vi "main.vi"() -> ()   [LabVIEW 2023]
uses:
  <vilib>/vision/Image Controls.llb/IMAQ Image.ctl
  <vilib>/vision/NI_Vision_Development_Module.lvlib
  <vilib>/vision/Pattern Matching.llb/IMAQ Match Range Setting.ctl
  <vilib>/vision/Shape Detection.llb/ShapeDetectionMatchOptions.ctl
  <vilib>/addons/database/NI_Database_API.lvlib
  <vilib>/addons/database/Command.llb/Cmd Set Parameter Value (C).vi
  <vilib>/addons/database/Command.llb/Cmd Delete.vi
  <vilib>/addons/database/Recordset.llb/Rec Destroy - Command.vi
  <vilib>/addons/database/Command.llb/Cmd Execute.vi
  <vilib>/addons/database/Connection.llb/DB Tools Open Connec (String).vi
  <vilib>/Utility/error.llb/DialogType.ctl
panel:
  in  "Python":bool
  out "Triangles":i32
  out "String":string
  out "Rectangles":i32
  out "Circles":i32
  out "Obraz":T1(plugin-control)
  in  "Output Path":path
  in  "Input Path":path=path "C:/Users/kacpe/Desktop/OSP/testp.png"
  in  "Refresh Button":bool
  in  "Process Stop Button":bool
  in  "Save As Button":bool
  in  "Labview":bool
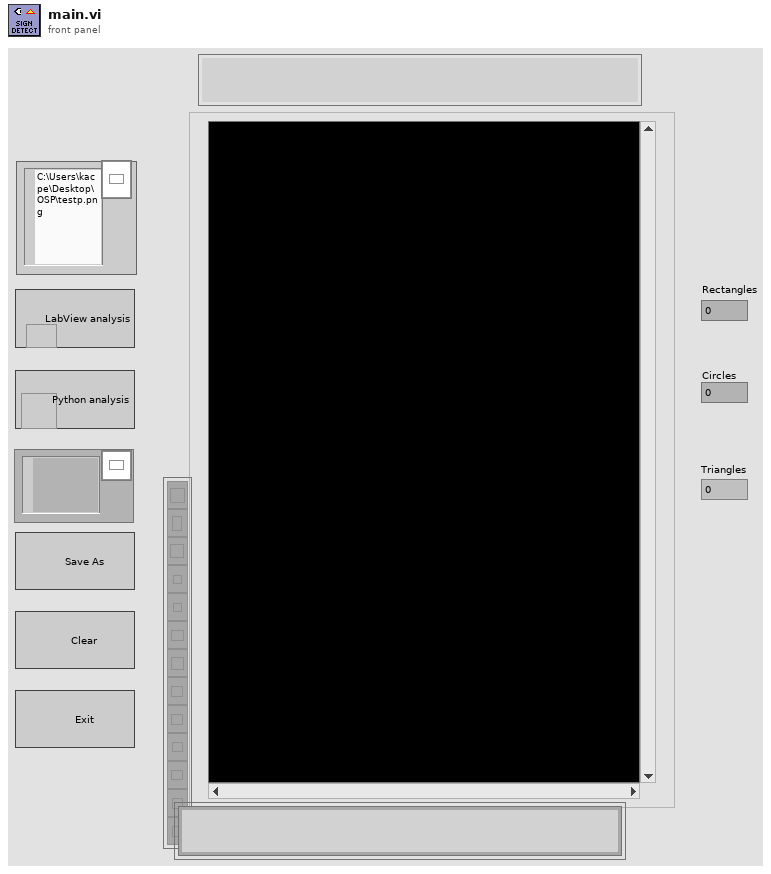
[diagram p1: front panel]
types:
  T1 = typedef "IMAQ Image.ctl" = refnum<image>
  T2 = enum32{"Invalid", "Standard", "Closed", "Hidden", "Minimized", "Maximized"}
  T3 = enum32{"invalid app kind", "Development System", "Run Time System", "Student Edition", "Embedded LabVIEW", "Evaluation", "Custom"}
  T4 = cluster{"Position":cluster{"x":sgl, "y":sgl}, "Angle":sgl, "Scale":sgl, "Score":sgl, "Bounding Box":cluster{"x":sgl, "y":sgl}[]}[]
  T5 = cluster{"Left":i32, "Top":i32, "Right":i32, "Bottom":i32}
  T6 = cluster{"Corners":cluster{"X":sgl, "Y":sgl}[], "Angle":dbl, "Width":dbl, "Height":dbl, "Score":dbl}[]
  T7 = cluster{"Position":cluster{"X":sgl, "Y":sgl}, "Radius":dbl, "Score":dbl}[]
  T8 = cluster{"Min Width":dbl, "Max Width":dbl, "Min Height":dbl, "Max Height":dbl}
  T9 = cluster{"Core":cluster{"Current VI Reference":refnum<vi>, "Close Panel on Exit?":bool}, "Obraz":T1, enum16{"null", "kwadrat", "kolo", "trojkat"}, "Rectangles":cluster{"Corners":cluster{"X":sgl, "Y":sgl}[], "Angle":dbl, "Width":dbl, "Height":dbl, "Score":dbl}[], "Circles":cluster{"Position":cluster{"X":sgl, "Y":sgl}, "Radius":dbl, "Score":dbl}[], "Triangle":cluster{"Position":cluster{"x":sgl, "y":sgl}, "Angle":sgl, "Scale":sgl, "Score":sgl, "Bounding Box":cluster{"x":sgl, "y":sgl}[]}[], "Znak":string, "Input Path":path, "Python cords":cluster{"Left":i32, "Top":i32, "Right":i32, "Bottom":i32}, "L/p":string}
  T10 = typedef "DialogType.ctl" = u16
  T11 = cluster{"Current VI Reference":refnum<vi>, "Close Panel on Exit?":bool}
  T12 = typedef "ShapeDetectionMatchOptions.ctl" = cluster{"Rotation":bool, "Scale":bool, "Occlusion":bool, "Range Settings":T13[]}
  T13 = typedef "IMAQ Match Range Setting.ctl" = cluster{"Match Constraints":u32, "Min":dbl, "Max":dbl}
  T14 = typedef "Image Type" = u32
  T15 = typedef "NI_Database_API.lvlib/Conn ObjectReference.ctl" = refnum<k1>
  T16 = typedef "NI_Database_API.lvlib/Cmd ObjectReference.ctl" = refnum<k1>
  T17 = typedef "NI_Database_API.lvlib/Cmd-Rec Object Reference.ctl" = refnum<k1>
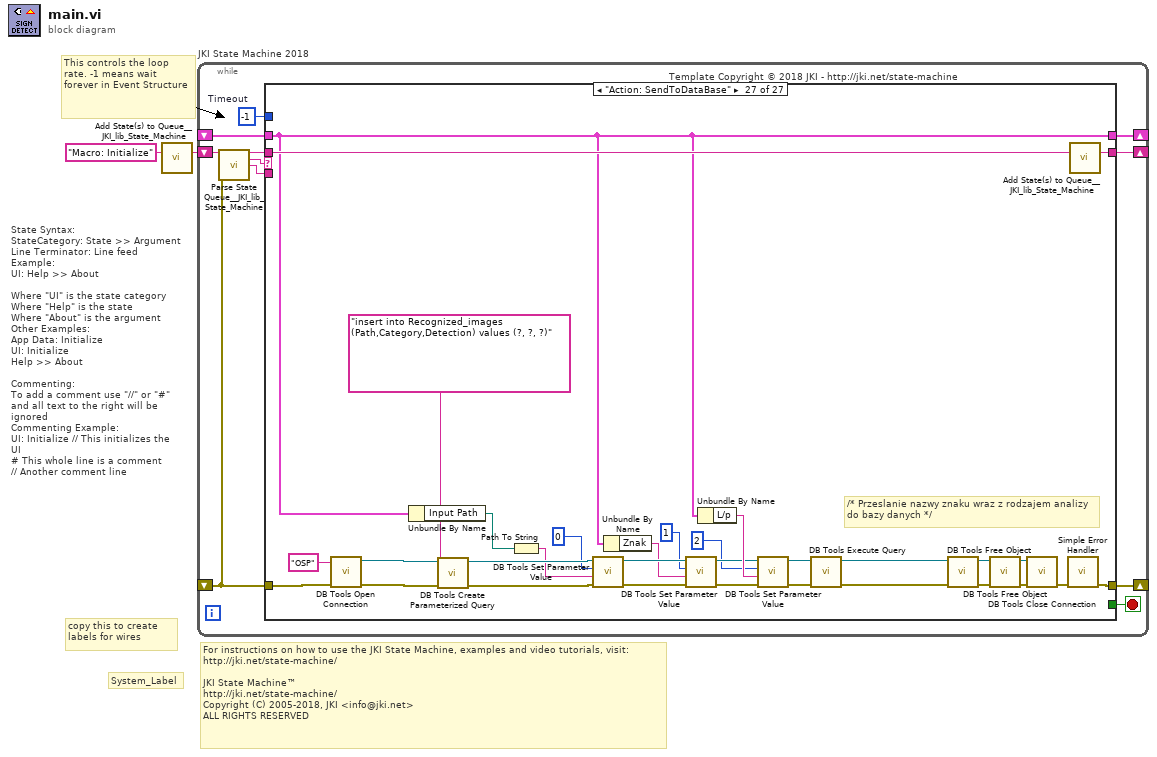
[diagram p0: block diagram]
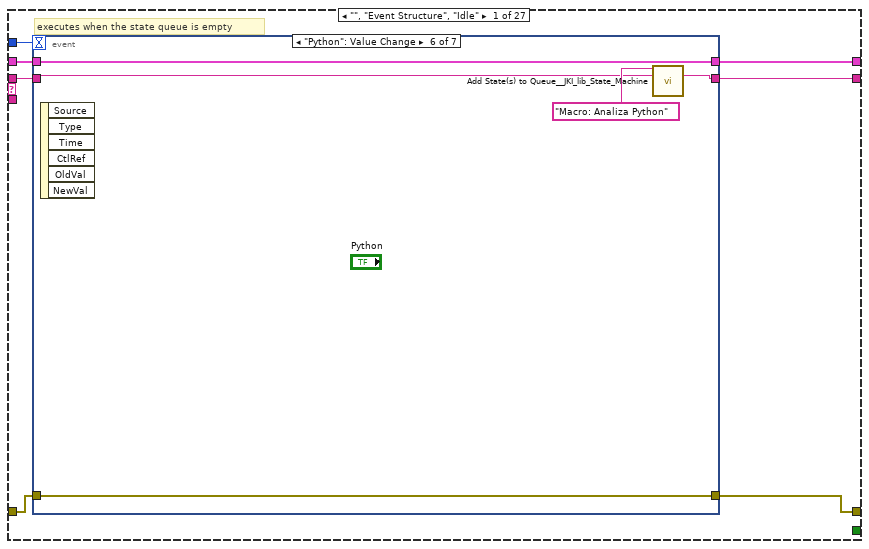
[diagram p2: hidden frame]
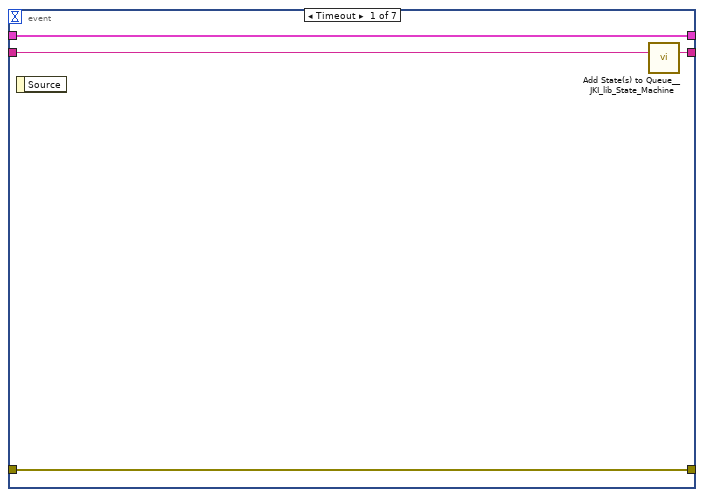
[diagram p3: hidden frame]
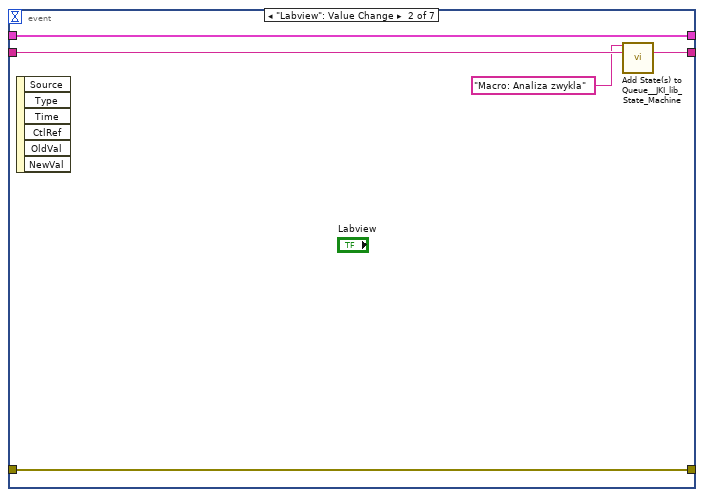
[diagram p4: hidden frame]
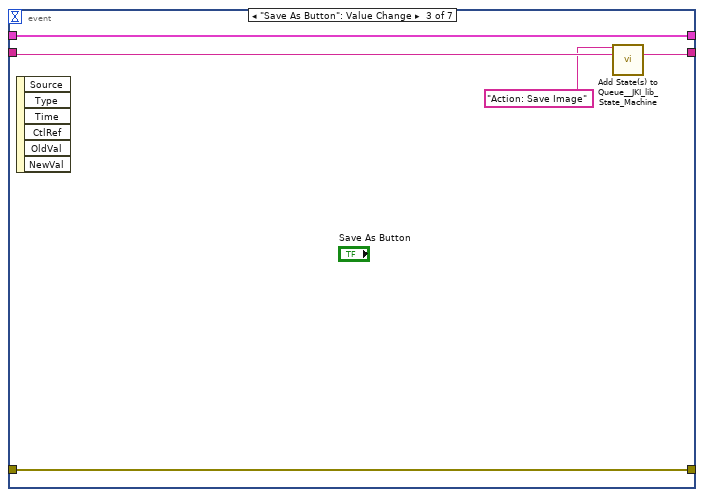
[diagram p5: hidden frame]
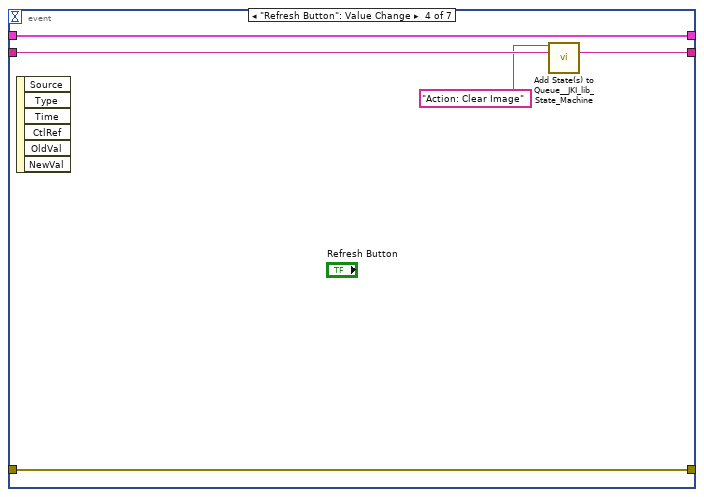
[diagram p6: hidden frame]
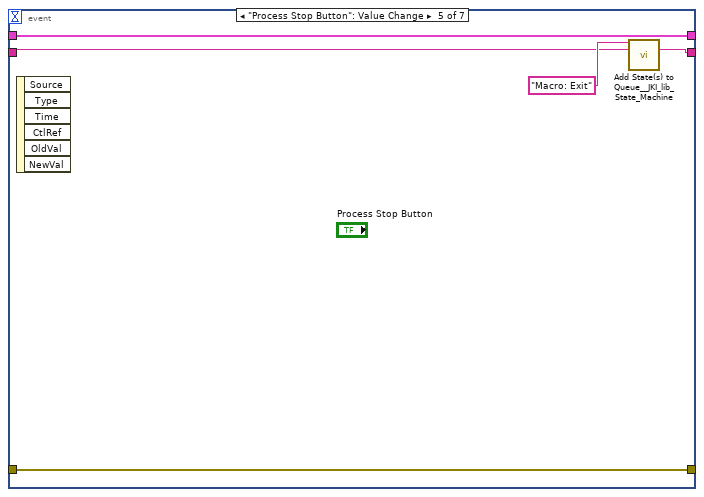
[diagram p7: hidden frame]
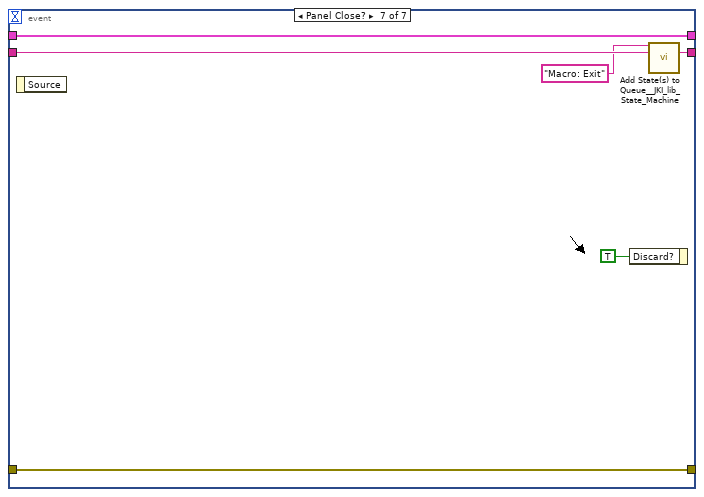
[diagram p8: hidden frame]
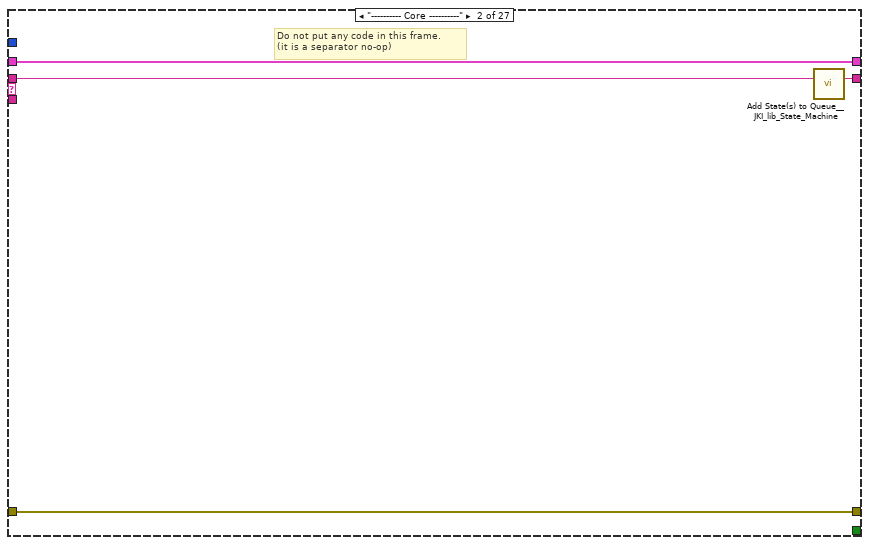
[diagram p9: hidden frame]
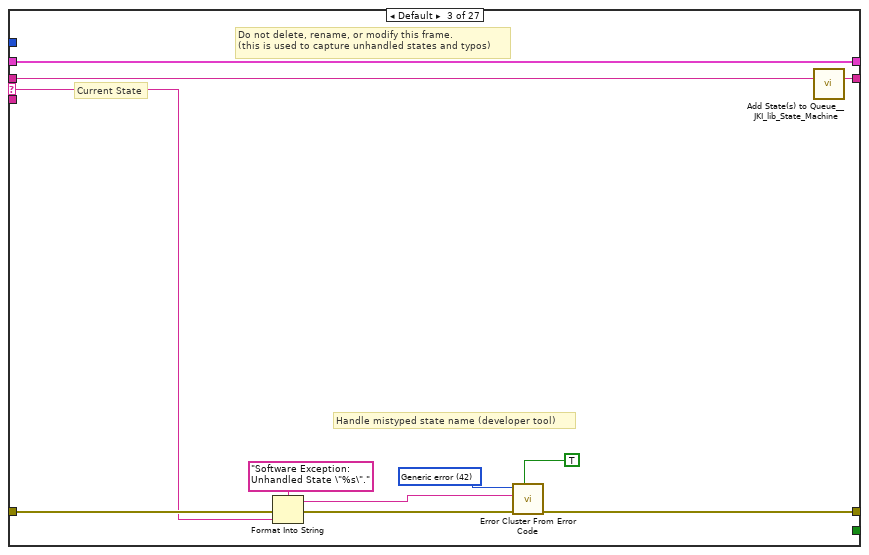
[diagram p10: hidden frame]
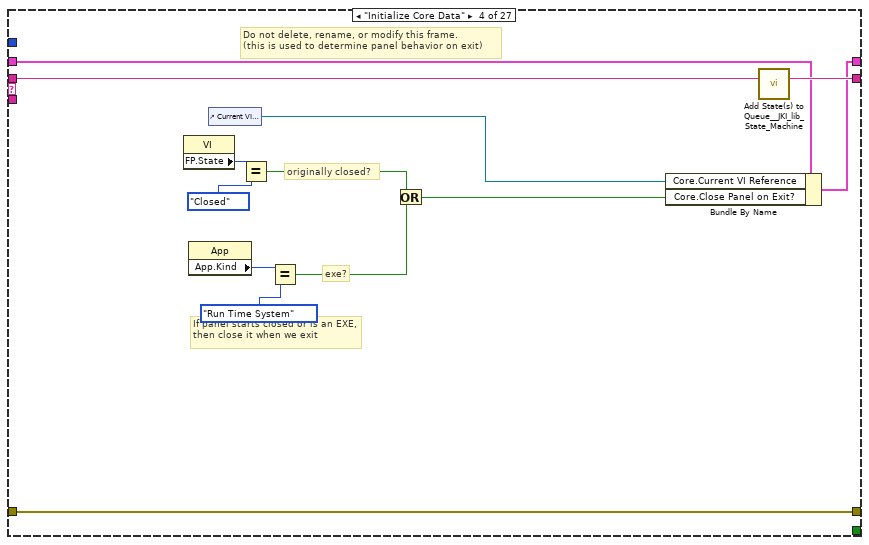
[diagram p11: hidden frame]
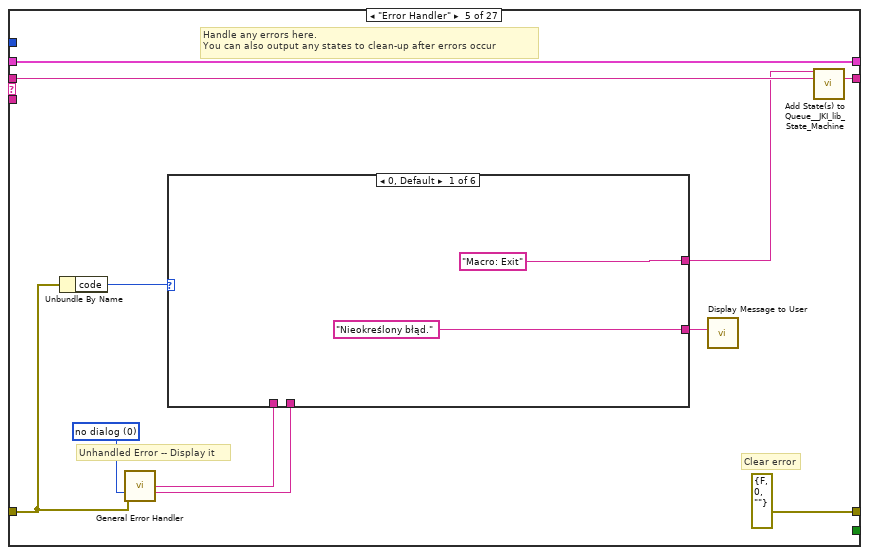
[diagram p12: hidden frame]
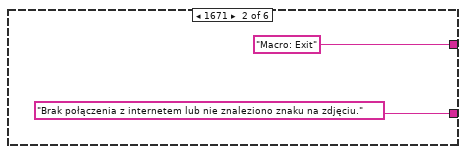
[diagram p13: hidden frame]
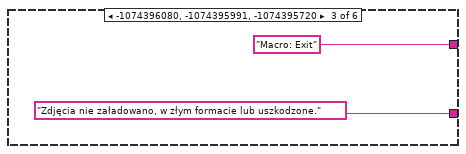
[diagram p14: hidden frame]
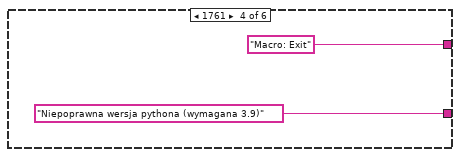
[diagram p15: hidden frame]
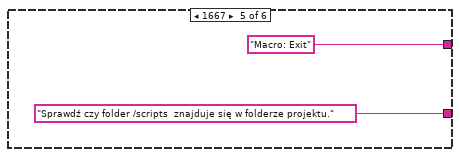
[diagram p16: hidden frame]
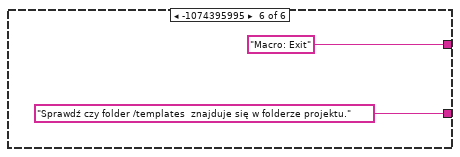
[diagram p17: hidden frame]
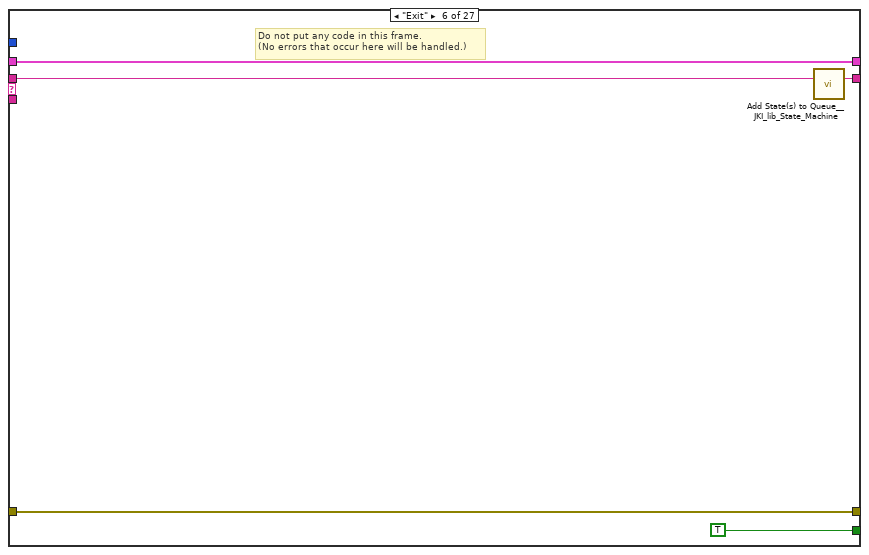
[diagram p18: hidden frame]
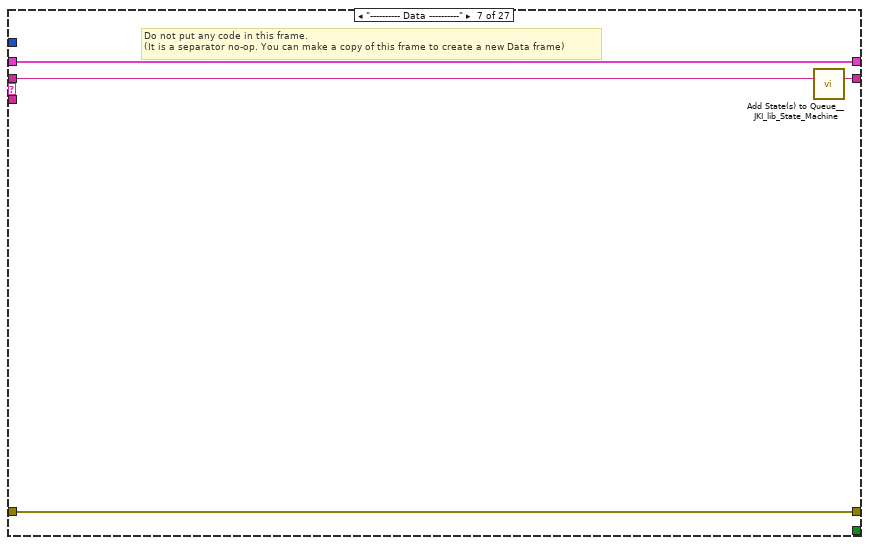
[diagram p19: hidden frame]
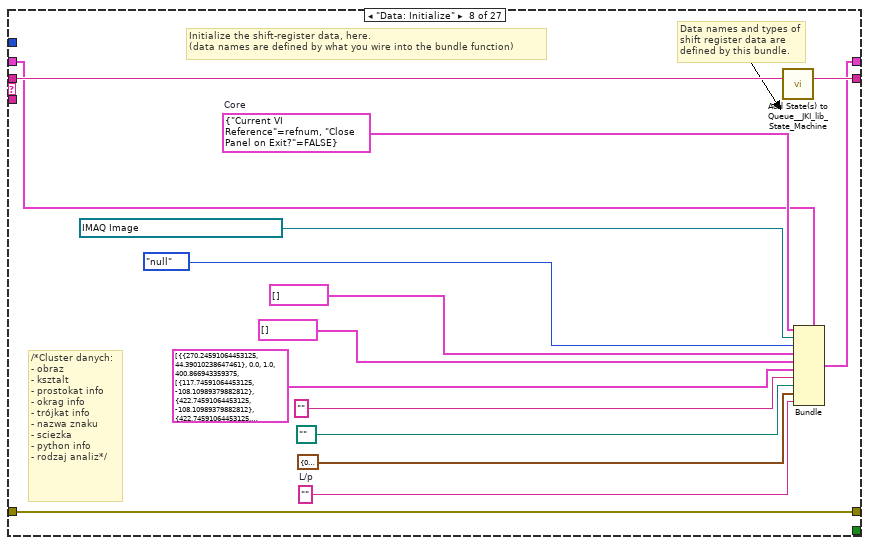
[diagram p20: hidden frame]
diagram:
  # "For instructions on how to use the JKI State Machine, examples and video tutorials, visit:\nhttp://jki.net/state-machine/\n\nJKI State Machine™\nhttp://jki.net/state-machine/\nCopyright (C) 2005-2018, JKI <info@jki.net>\nALL RIGHTS RESERVED"
  # "State Syntax:\nStateCategory: State >> Argument\nLine Terminator: Line feed\nExample:\nUI: Help >> About\n\nWhere \"UI\" is the state category\nWhere \"Help\" is the state\nWhere \"About\" is the argument\nOther Examples:\nApp Data: Initialize\nUI: Initialize\nHelp >> About\n\nCommenting:\nTo add a comment use \"//\" or \"#\" and all text to the right will be ignored\nCommenting Example:\nUI: Initialize // This initializes the UI\n# This whole line is a comment\n// Another comment line"
  # "copy this to create labels for wires"
  # "This controls the loop rate. -1 means wait forever in Event Structure"
  # "System_Label"
  n1 = call <vilib>:"Add State(s) to Queue__JKI_lib_State_Machine.vi"("State(s) in (\"\")"="Macro: Initialize") -> ("States Out"=w2:string)  [unwired: 14 in]
  n2 = while "JKI State Machine 2018" {
    shift-right: [w6] -> _
    shift-left: _ -> [w5]
    shift-right: [w9] -> _
    shift-left: _ -> [w3]
    shift-right: [w8] -> _
    shift-left: w2 -> [w10]
    stop <- w7 stop-if-true
    w4 = -1  # Timeout
    # "Template Copyright © 2018 JKI - http://jki.net/state-machine"
    n3 = call <vilib>:"Parse State Queue__JKI_lib_State_Machine.vi"("State Queue"=w10, "Error In (no error)"=w3) -> ("Remaining States"=w12:string, "Current State"=w13:string, "Arguments"=w11:string)  [unwired: 11 in]
    n4 = case shown="\"Action: SendToDataBase\"" w13 {
      selector: w13 -> [_ _ w60 _ _ _ _ _ _ _ _ _ _ _ _ _ _ _ _ _ _ _ _ _ _ _ _]
      tunnel: w12 -> [w20 w59 w64 w83 w94 w111 w115 w130 w136 w140 w144 w149 w155 w166 w230 w235 w240 w245 w255 w259 w298 w313 w344 w354 w361 w369 w400]
      tunnel: w11 -> [_ _ _ _ _ _ _ _ _ _ _ _ w150 w161 _ _ _ _ _ _ _ _ _ _ _ _ _]
      tunnel: w5 -> [w18 w56 w62 w72 w91 w109 w112 w119 w132 w137 w143 w147 w153 w160 w227 w232 w237 w242 w247 w256 w287 w307 w327 w346 w356 w364 w381]
      tunnel: [w17 w57 w66 w81 errorcluster {"status"=FALSE, "code"=0, "source"=""} ("error out") w108 w113 w128 w133 w138 w145 w146 w151 w163 w228 w233 w238 w243 w253 w257 w265 w311 w342 w349 w359 w367 w374] -> w9
      tunnel: w3 -> [w16 w57 w65 w81 w87 w108 w113 w128 w134 w138 w145 w146 w152 w164 w228 w233 w238 w243 w253 w257 w291 w310 w341 w349 w358 w367 w373]
      tunnel: [w19 w58 w63 w82 w93 w110 w114 w129 w135 w139 w144 w148 w154 w165 w229 w234 w239 w244 w254 w258 w298 w312 w343 w353 w360 w368 w399] -> w8
      tunnel: [_ _ _ _ _ TRUE _ _ _ _ _ _ _ _ _ _ _ _ _ _ _ _ _ _ _ _ _] -> w7
      tunnel: [w15 w56 w62 w71 w91 w109 w112 w118 w132 w137 w143 w147 w153 w160 w227 w232 w237 w242 w247 w256 w288 w308 w328 w347 w356 w365 w381] -> w6
      tunnel: w4 -> [w14 _ _ _ _ _ _ _ _ _ _ _ _ _ _ _ _ _ _ _ _ _ _ _ _ _ _]
      frame "", "Event Structure", "Idle" {
        # "executes when the state queue is empty"
        n5 = event shown="[5] \"Python\": Value Change" {
          selector: _ -> [_ _ _ _ _ _ _]
          dyn-events: _ -> [_ _ _ _ _ _ _]
          timeout: w14 -> [_ _ _ _ _ _ _]
          tunnel: w20 -> [w24 w27 w31 w36 w41 w46 w55]
          tunnel: [w23 w28 w32 w37 w43 w48 w54] -> w19
          tunnel: w18 -> [w21 w29 w34 w39 w44 w49 w52]
          tunnel: [w22 w25 w33 w38 w40 w45 w53] -> w17
          tunnel: w16 -> [w22 w25 w33 w38 w40 w45 w53]
          tunnel: [w21 w29 w34 w39 w44 w49 w52] -> w15
          event Timeout {
            n6 = event-data() -> ()  [unwired: 1 in, 1 out]
            n7 = call <vilib>:"Add State(s) to Queue__JKI_lib_State_Machine.vi"("State(s) in (\"\")"=w24) -> ("States Out"=w23:string)  [unwired: 14 in]
          }
          event "Labview": Value Change {
            n8 = event-data() -> ()  [unwired: 1 in, 6 out]
            n9 = call <vilib>:"Add State(s) to Queue__JKI_lib_State_Machine.vi"("State(s) in Front (\"\")"="Macro: Analiza zwykla" ("State(s) in Front (\"\")"), "State(s) in (\"\")"=w27) -> ("States Out"=w28:string)  [unwired: 13 in]
          }
          event "Save As Button": Value Change {
            n10 = event-data() -> ()  [unwired: 1 in, 6 out]
            n11 = call <vilib>:"Add State(s) to Queue__JKI_lib_State_Machine.vi"("State(s) in Front (\"\")"="Action: Save Image" ("State(s) in Front (\"\")"), "State(s) in (\"\")"=w31) -> ("States Out"=w32:string)  [unwired: 13 in]
          }
          event "Refresh Button": Value Change {
            n12 = event-data() -> ()  [unwired: 1 in, 6 out]
            n13 = call <vilib>:"Add State(s) to Queue__JKI_lib_State_Machine.vi"("State(s) in Front (\"\")"="Action: Clear Image" ("State(s) in Front (\"\")"), "State(s) in (\"\")"=w36) -> ("States Out"=w37:string)  [unwired: 13 in]
          }
          event "Process Stop Button": Value Change {
            n14 = event-data() -> ()  [unwired: 1 in, 6 out]
            n15 = call <vilib>:"Add State(s) to Queue__JKI_lib_State_Machine.vi"("State(s) in Front (\"\")"="Macro: Exit", "State(s) in (\"\")"=w41) -> ("States Out"=w43:string)  [unwired: 13 in]
          }
          event "Python": Value Change {
            n16 = event-data() -> ()  [unwired: 1 in, 6 out]
            n17 = call <vilib>:"Add State(s) to Queue__JKI_lib_State_Machine.vi"("State(s) in Front (\"\")"="Macro: Analiza Python", "State(s) in (\"\")"=w46) -> ("States Out"=w48:string)  [unwired: 13 in]
          }
          event Panel Close? {
            n18 = event-data() -> ()  [unwired: 1 in, 1 out]
            n19 = event-data ("Event Filter Node")("Discard?"=TRUE) -> ()  [unwired: 1 in, 1 out]
            n20 = call <vilib>:"Add State(s) to Queue__JKI_lib_State_Machine.vi"("State(s) in Front (\"\")"="Macro: Exit", "State(s) in (\"\")"=w55) -> ("States Out"=w54:string)  [unwired: 13 in]
          }
        }
      }
      frame "---------- Core ----------" {
        # "Do not put any code in this frame.\n(it is a separator no-op)"
        n21 = call <vilib>:"Add State(s) to Queue__JKI_lib_State_Machine.vi"("State(s) in (\"\")"=w59) -> ("States Out"=w58:string)  [unwired: 14 in]
      }
      frame Default {
        w69 = 42 items=["No error", "Argument error", "Memory is full", "Out of zone", "End of file", "File already open", "Generic file I/O error", "File not found", "File permission error", "Disk is full", "Duplicate path", "Too many files open", "System feature not enabled", "Resource file not found", "Cannot add resource", "Resource not found", "Image not found", "Image memory error", "Pen does not exist", "Config type invalid", "Config token not found", "Config parse error", "Config memory error", "Bad external code format", "Bad external code offset", "External code not present", "Null window", "Destroy window error", "Null menu", "Print aborted", "Bad print record", "Print driver error", "Windows error during printing", "Memory error during printing", "Print dialog error", "Generic print error", "Invalid device refnum", "Device not found", "Device parameter error", "Device unit error", "Cannot open device", "Device call aborted", "Generic error", "Cancelled by user", "Object ID too low", "Object ID too high", "Object not in heap", "Unknown heap", "Unknown object (invalid DefProc)", "Unknown object (DefProc not in table)", "Message out of range", "Invalid (null) method", "Unknown message", "Manager call not supported", "Bad address", "Network operation in progress", "Network operation timed out", "Connection is busy", "Network attribute not supported", "Network error", "Address in use", "System out of memory", "Connection aborted", "Connection refused", "Not connected", "Already connected", "Connection closed", "Initialization error (interapplication manager)", "Bad occurrence", "Wait on unbound occurrence handler", "Occurrence queue overflow", "Datalog type conflict", "Unused", "Unrecognized type (interapplication manager)", "Memory corrupt", "Failed to make temporary DLL", "Old CIN version", "Drag socket not found", "Failed to load drop-object", "Failed to register OLE object", "Failed to release OLE object", "Format specifier type mismatch", "Unknown format specifier", "Too few format specifiers", "Too many format specifiers", "Scan failed", "Newer CIN version", "Error converting to variant", "Runtime menu error", "Password tampered", "Variant attribute not found", "Incompatible variant data type", "Event data is not available", "Event Store is not present", "Occurrence is not found", "Event Queue is not created", "Event info is not available", "Refnum passed is NULL", "Error retrieving Class GUID", "Error retrieving CoClass GUID", "Error retrieving TypeLib GUID.", "Bad built application magic bytes.", "Specific driver is different from the specific driver associated with the Logical Name.", "There is no session opened to the class driver.", "Max Error", "MAX - Error with config objects", "MAX - Error loading configuration", "MAX - Group not supported"]
        # "Current State"
        # "Do not delete, rename, or modify this frame.\n(this is used to capture unhandled states and typos)"
        # "Handle mistyped state name (developer tool)"
        n22 = Format Into String(format string="Software Exception: Unhandled State \"%s\"." ("message"), error in=w65, w60) -> (resulting string=w68:string, error out=w67:errorcluster)  [unwired: 1 in]
        n23 = call <vilib>:"Error Cluster From Error Code.vi"("show call chain? (False)"=TRUE, "error in (no error)"=w67, "error message (\"\")"=w68, "error code (0)"=w69) -> ("error out"=w66:errorcluster)  [unwired: 5 in]
        n24 = call <vilib>:"Add State(s) to Queue__JKI_lib_State_Machine.vi"("State(s) in (\"\")"=w64) -> ("States Out"=w63:string)  [unwired: 14 in]
      }
      frame "Initialize Core Data" {
        # "Do not delete, rename, or modify this frame.\n(this is used to determine panel behavior on exit)"
        # "originally closed?"
        # "exe?"
        # "If panel starts closed or is an EXE, then close it when we exit"
        n25 = property on="Property Node" class="VI"() -> ("FP.State"=w75:T2)  [unwired: 2 in, 2 out]
        n26 = property on="Property Node" class="App"() -> ("App.Kind"=w80:T3)  [unwired: 2 in, 2 out]
        n27 = control-ref of="Current VI Reference"() -> (w76:refnum<vi>)
        n28 = Equal?(x=w75, y=T2."Closed" ("Front Panel Window:State")) -> (x = y?=w73:bool)
        n29 = Equal?(x=w80, y=T3."Run Time System" ("Application:Kind")) -> (x = y?=w78:bool)
        n30 = Or(x=w73, y=w78) -> (x .or. y?=w77:bool)
        n31 = Bundle By Name(cluster=w72, "Core.Current VI Reference"=w76, "Core.Close Panel on Exit?"=w77) -> (w71:T9)
        n32 = call <vilib>:"Add State(s) to Queue__JKI_lib_State_Machine.vi"("State(s) in (\"\")"=w83) -> ("States Out"=w82:string)  [unwired: 14 in]
      }
      frame "Error Handler" {
        w84 = T10 0 items=["no dialog", "OK message", "continue or stop message", "OK message + warnings", "continue/stop + warnings"] ("type of dialog (OK msg:1)")
        # "Unhandled Error -- Display it"
        # "Handle any errors here.\nYou can also output any states to clean-up after errors occur"
        # "Clear error"
        n33 = Unbundle By Name(w87) -> ("code"=w90:i32)
        n34 = call <vilib>:"General Error Handler.vi"("type of dialog (OK msg:1)"=w84, "error in (no error)"=w87) -> ("source out"=w85:string, "message"=w86:string)  [unwired: 9 in, 3 out]
        n35 = case shown="0, Default" w90 {
          tunnel: ["Macro: Exit" "Macro: Exit" "Macro: Exit" "Macro: Exit" "Macro: Exit" "Macro: Exit"] -> w89
          tunnel: ["Nieokreślony błąd." "Brak połączenia z internetem lub nie znaleziono znaku na zdjęciu." "Zdjęcia nie załadowano, w złym formacie lub uszkodzone." "Niepoprawna wersja pythona (wymagana 3.9)" "Sprawdź czy folder /scripts  znajduje się w folderze projektu." "Sprawdź czy folder /templates  znajduje się w folderze projektu."] -> w88
          tunnel: w86 -> [_ _ _ _ _ _]
          tunnel: w85 -> [_ _ _ _ _ _]
          frame 0, Default {
          }
          frame 1671 {
          }
          frame -1074396080, -1074395991, -1074395720 {
          }
          frame 1761 {
          }
          frame 1667 {
          }
          frame -1074395995 {
          }
        }
        n36 = call "Display Message to User"("Message"=w88) -> ()  [unwired: 9 in, 2 out]
        n37 = call <vilib>:"Add State(s) to Queue__JKI_lib_State_Machine.vi"("State(s) in Front (\"\")"=w89, "State(s) in (\"\")"=w94) -> ("States Out"=w93:string)  [unwired: 13 in]
      }
      frame "Exit" {
        # "Do not put any code in this frame.\n(No errors that occur here will be handled.)"
        n38 = call <vilib>:"Add State(s) to Queue__JKI_lib_State_Machine.vi"("State(s) in (\"\")"=w111) -> ("States Out"=w110:string)  [unwired: 14 in]
      }
      frame "---------- Data ----------" {
        # "Do not put any code in this frame.\n(It is a separator no-op. You can make a copy of this frame to create a new Data frame)"
        n39 = call <vilib>:"Add State(s) to Queue__JKI_lib_State_Machine.vi"("State(s) in (\"\")"=w115) -> ("States Out"=w114:string)  [unwired: 14 in]
      }
      frame "Data: Initialize" {
        w116 = ""  # L/p
        w127 = T11 {"Current VI Reference"=refnum, "Close Panel on Exit?"=FALSE}  # Core
        # "/*Cluster danych:\n- obraz\n- ksztalt\n- prostokat info\n- okrag info\n- trójkat info\n- nazwa znaku\n- sciezka\n- python info\n- rodzaj analiz*/"
        # "Data names and types of shift register data are defined by this bundle."
        # "Initialize the shift-register data, here.\n(data names are defined by what you wire into the bundle function)"
        n40 = call <vilib>:"Add State(s) to Queue__JKI_lib_State_Machine.vi"("State(s) in (\"\")"=w130) -> ("States Out"=w129:string)  [unwired: 14 in]
        n41 = Bundle(cluster=w119, "Core"=w127, "Obraz"=T1 refnum, enum16{"null", "kwadrat", "kolo", "trojkat"}."null", "Rectangles"=T6 [], "Circles"=T7 [], "Triangle"=T4 [{"Position"={"x"=270.2459, "y"=44.390102}, "Angle"=0.0, "Scale"=1.0, "Score"=400.86694, "Bounding Box"=[{"x"=117.74591, "y"=-108.10989}, {"x"=422.7459, "y"=-108.10989}, {"x"=422.7459, "y"=196.8901}, {"x"=117.74591, "y"=196.8901}, {"x"=117.74591, "y"=-108.10989}]}], "Znak"="", "Input Path"=path "", "Python cords"=T5 {"Left"=0, "Top"=0, "Right"=0, "Bottom"=0}, "L/p"=w116) -> (w118:T9)
      }
      frame "Data: Cleanup" {
        # "Cleanup any data and references, here.\n(this is called automatically, by the Macro: Exit)"
        n42 = Unbundle By Name(w132) -> ("Core.Current VI Reference"=w131:refnum<vi>)
        n43 = Close Reference(reference=w131, error in (no error)=w134) -> (error out=w133:errorcluster)
        n44 = call <vilib>:"Add State(s) to Queue__JKI_lib_State_Machine.vi"("State(s) in (\"\")"=w136) -> ("States Out"=w135:string)  [unwired: 14 in]
      }
      frame "---------- UI ----------" {
        # "Do not put any code in this frame.\n(It is a separator no-op. You can make a copy of this frame to create a new UI frame)"
        n45 = call <vilib>:"Add State(s) to Queue__JKI_lib_State_Machine.vi"("State(s) in (\"\")"=w140) -> ("States Out"=w139:string)  [unwired: 14 in]
      }
      frame "UI: Update" {
        # "/* Aktualizacja obrazu oraz nazwy znaku \nna front panelu */"
        n46 = Unbundle By Name(w143) -> ("Obraz"=→"Obraz":T1, "Znak"=→"String":string)
      }
      frame "UI: Initialize" {
        # "Initialize the User Interface, here.\n(this is called automatically, by the Macro: Init)"
        n47 = call <vilib>:"Add State(s) to Queue__JKI_lib_State_Machine.vi"("State(s) in (\"\")"=w149) -> ("States Out"=w148:string)  [unwired: 14 in]
      }
      frame "UI: Cursor Set" {
        # "Argument"
        # "Set and Unset Cursor Busy.\n(Usage: \"UI: Cursor Set >> Busy|Idle\")"
        n48 = case shown="\"Idle\", Default" w150 {
          tunnel: w152 -> [w157 w159]
          tunnel: [w156 w158] -> w151
          frame "Idle", Default {
            n49 = call <vilib>:"Unset Busy.vi"("error in (no error)"=w157) -> ("error out"=w156:errorcluster)  [unwired: 10 in]
          }
          frame "Busy" {
            n50 = call <vilib>:"Set Busy.vi"("error in (no error)"=w159) -> ("error out"=w158:errorcluster)  [unwired: 9 in, 1 out]
          }
        }
        n51 = call <vilib>:"Add State(s) to Queue__JKI_lib_State_Machine.vi"("State(s) in (\"\")"=w155) -> ("States Out"=w154:string)  [unwired: 14 in]
      }
      frame "UI: Front Panel State" {
        # "Argument"
        # "Set Front Panel Open or Closed\n(Usage: \"UI: Front Panel State >> Open|Close\")"
        n52 = Unbundle By Name(w160) -> ("Core.Current VI Reference"=w162:refnum<vi>)
        n53 = case shown="\"Open\", \"Standard\", Default" w161 {
          tunnel: w164 -> [w172 w185 w196 w208 w220]
          tunnel: [w173 w186 w197 w209 w221] -> w163
          tunnel: w162 -> [_ _ _ _ _]
          frame "Open", "Standard", Default {
            w167 = T2."Standard" ("State")
            n54 = property on="Property Node" class="VI"(error in=w172) -> (reference out=w170:refnum<vi>, error out=w171:errorcluster, "FP.State"=w169:T2)  [unwired: 1 in]
            n55 = Not Equal?(x=w169, y=w167) -> (x != y?=w168:bool)
            n56 = case shown="False" w168 {
              tunnel: [w177 w179] -> w173
              tunnel: w171 -> [w176 w179]
              tunnel: w170 -> [w175 _]
              tunnel: w167 -> [w174 _]
              frame True {
                n57 = invoke on="Invoke Node" class="VI" method="FP.Open"(reference=w175, error in=w176, "Activate"=TRUE, "State"=w174) -> (error out=w177:errorcluster)  [unwired: 1 in, 4 out]
              }
              frame False {
              }
            }
          }
          frame "Close", "Closed" {
            n58 = property on="Property Node" class="VI"(error in=w185) -> (reference out=w183:refnum<vi>, error out=w184:errorcluster, "FP.State"=w181:T2)  [unwired: 1 in]
            n59 = Not Equal?(x=w181, y=T2."Closed" ("Front Panel Window:State")) -> (x != y?=w180:bool)
            n60 = case shown="True" w180 {
              tunnel: [w187 w190] -> w186
              tunnel: w184 -> [w187 w189]
              tunnel: w183 -> [_ w188]
              frame False {
              }
              frame True {
                n61 = invoke on="Invoke Node" class="VI" method="FP.Close"(reference=w188, error in=w189) -> (error out=w190:errorcluster)  [unwired: 1 in, 2 out]
              }
            }
          }
          frame "Hidden", "Hide" {
            w191 = T2."Hidden" ("State")
            n62 = property on="Property Node" class="VI"(error in=w196) -> (reference out=w194:refnum<vi>, error out=w195:errorcluster, "FP.State"=w193:T2)  [unwired: 1 in]
            n63 = Not Equal?(x=w193, y=w191) -> (x != y?=w192:bool)
            n64 = case shown="True" w192 {
              tunnel: [w201 w202] -> w197
              tunnel: w195 -> [w200 w202]
              tunnel: w194 -> [w199 _]
              tunnel: w191 -> [w198 _]
              frame True {
                n65 = invoke on="Invoke Node" class="VI" method="FP.Open"(reference=w199, error in=w200, "State"=w198) -> (error out=w201:errorcluster)  [unwired: 2 in, 4 out]
              }
              frame False {
              }
            }
          }
          frame "Minimize", "Minimized" {
            w203 = T2."Minimized" ("State")
            n66 = property on="Property Node" class="VI"(error in=w208) -> (reference out=w206:refnum<vi>, error out=w207:errorcluster, "FP.State"=w205:T2)  [unwired: 1 in]
            n67 = Not Equal?(x=w205, y=w203) -> (x != y?=w204:bool)
            n68 = case shown="True" w204 {
              tunnel: [w213 w214] -> w209
              tunnel: w207 -> [w212 w214]
              tunnel: w206 -> [w211 _]
              tunnel: w203 -> [w210 _]
              frame True {
                n69 = invoke on="Invoke Node" class="VI" method="FP.Open"(reference=w211, error in=w212, "State"=w210) -> (error out=w213:errorcluster)  [unwired: 2 in, 4 out]
              }
              frame False {
              }
            }
          }
          frame "Maximize", "Maximized" {
            w215 = T2."Maximized" ("State")
            n70 = property on="Property Node" class="VI"(error in=w220) -> (reference out=w218:refnum<vi>, error out=w219:errorcluster, "FP.State"=w217:T2)  [unwired: 1 in]
            n71 = Not Equal?(x=w217, y=w215) -> (x != y?=w216:bool)
            n72 = case shown="True" w216 {
              tunnel: [w225 w226] -> w221
              tunnel: w219 -> [w224 w226]
              tunnel: w218 -> [w223 _]
              tunnel: w215 -> [w222 _]
              frame True {
                n73 = invoke on="Invoke Node" class="VI" method="FP.Open"(reference=w223, error in=w224, "State"=w222) -> (error out=w225:errorcluster)  [unwired: 2 in, 4 out]
              }
              frame False {
              }
            }
          }
        }
        n74 = call <vilib>:"Add State(s) to Queue__JKI_lib_State_Machine.vi"("State(s) in (\"\")"=w166) -> ("States Out"=w165:string)  [unwired: 14 in]
      }
      frame "---------- Macro ----------" {
        # "Do not put any code in this frame.\n(It is a separator no-op. You can make a copy of this frame to create a new Macro frame)"
        n75 = call <vilib>:"Add State(s) to Queue__JKI_lib_State_Machine.vi"("State(s) in (\"\")"=w230) -> ("States Out"=w229:string)  [unwired: 14 in]
      }
      frame "Macro: Initialize" {
        w231 = "Data: Initialize\nInitialize Core Data\nUI: Initialize\nUI: Front Panel State >> Open"  # Data: Initialize Initialize Core Data UI: Initialize UI: Front Panel State >> Open
        # "Initialization Macro\n(This is called once, when the VI starts)"
        n76 = call <vilib>:"Add State(s) to Queue__JKI_lib_State_Machine.vi"("State(s) in Front (\"\")"=w231, "State(s) in (\"\")"=w235) -> ("States Out"=w234:string)  [unwired: 13 in]
      }
      frame "Macro: Analiza Python" {
        # "/* Macro do anlizy z wykorzystaniem \nskryptu python */"
        # "Initialization Macro\n(This is called once, when the VI starts)"
        n77 = call <vilib>:"Add State(s) to Queue__JKI_lib_State_Machine.vi"("State(s) in Front (\"\")"="Action: Load Image\nAction: Python Analyze\nAction: Draw Boundling Box\nAction: SendToDataBase \nUI: Update", "State(s) in (\"\")"=w240) -> ("States Out"=w239:string)  [unwired: 13 in]
      }
      frame "Macro: Analiza zwykla" {
        # "/* Macro do anlizy z wykorzystaniem \nfunkcji LabView */"
        # "Initialization Macro\n(This is called once, when the VI starts)"
        n78 = call <vilib>:"Add State(s) to Queue__JKI_lib_State_Machine.vi"("State(s) in Front (\"\")"="Action: Load Image\nAction: Analyze Image\nAction: Draw Boundling Box\nAction: SendToDataBase \nUI: Update", "State(s) in (\"\")"=w245) -> ("States Out"=w244:string)  [unwired: 13 in]
      }
      frame "Macro: Exit" {
        # "Exit Macro\n(This is called once, when the VI exits)"
        n79 = Unbundle By Name(w247) -> ("Core.Close Panel on Exit?"=w246:bool)
        n80 = Select(t="UI: Front Panel State >> Close", s=w246, f="" ("Empty String Constant")) -> (s? t:f=w250:string)
        n81 = call <vilib>:"Add State(s) to Queue__JKI_lib_State_Machine.vi"("State(s) in (\"\")"=w250, "State(s) at Back (\"\")"="Data: Cleanup\nExit") -> ("States Out"=w248:string)  [unwired: 13 in]
        n82 = call <vilib>:"Add State(s) to Queue__JKI_lib_State_Machine.vi"("State(s) in Front (\"\")"=w248, "State(s) in (\"\")"=w255) -> ("States Out"=w254:string)  [unwired: 13 in]
      }
      frame "---------- Action ----------" {
        # "Template Separator\n(You can make a copy of, or modify, this frame)"
        n83 = call <vilib>:"Add State(s) to Queue__JKI_lib_State_Machine.vi"("State(s) in (\"\")"=w259) -> ("States Out"=w258:string)  [unwired: 14 in]
      }
      frame "Action: Python Analyze" {
        # "/* Analiza z wykorzystniem jezyka python:\nPobranie sciezki do zdjecia i wykorzystanie jej do dwoch skryptow, z czego jeden zwraca nazwa wykrytego znaku, a drugi wspolrzedne do wygenerowania ramki wokol znaku\nW wypadku innej wersji python zamienic 'Python Version' w obu skryptach. (zalecana wersja 3.9) */"
        n84 = Unbundle By Name(w287) -> ("Input Path"=w286:path)
        n85 = Open Python Session(python version="3.7" ("Python version"), 3:w291) -> (session out=w293:refnum<k35>, error out=w290:errorcluster)  [unwired: 1 in]
        n86 = call <vilib>:"Application Directory.vi"() -> ("Application Directory"=w297:path)
        n87 = Build Path(base path=w297, name or relative path="scripts\\name.py") -> (appended path=w285:path)
        n88 = Path To String(path=w286) -> (string=w275:string)
        n89 = node ("Python Node")(w293, w285, "Analyze" ("function name"), w290, w275, w275) -> (w292:refnum<k35>, w289:errorcluster, w281:string)  [unwired: 1 in, 2 out]
        n90 = Close Python Session(session in=w292, error in=w289) -> (11:w264:errorcluster)
        n91 = Open Python Session(python version="3.7" ("Python version"), 3:w264) -> (session out=w269:refnum<k35>, error out=w263:errorcluster)  [unwired: 1 in]
        n92 = call <vilib>:"Application Directory.vi"() -> ("Application Directory"=w280:path)
        n93 = Build Array(0.0) -> (w276:dbl[])
        n94 = Build Path(base path=w280, name or relative path="scripts\\cords.py") -> (appended path=w278:path)
        n95 = node ("Python Node")(w269, w278, "Analyze" ("function name"), w263, w276, w275) -> (w277:refnum<k35>, w262:errorcluster, w274:dbl[])  [unwired: 1 in, 2 out]
        n96 = Index Array(array=w274, index #1=0 ("index"), index #2=1 ("index"), index #3=2 ("index"), index #4=3 ("index")) -> (element #1=w261:dbl, element #2=w273:dbl, element #3=w272:dbl, element #4=w271:dbl)
        n97 = Bundle By Name(cluster=w287, "Znak"=w281, "Python cords.Left"=w261, "Python cords.Top"=w273, "Python cords.Right"=w272, "Python cords.Bottom"=w271, "L/p"="Python") -> (w288:T9)
        n98 = Close Python Session(session in=w277, error in=w262) -> (11:w265:errorcluster)
      }
      frame "Action: Draw Boundling Box" {
        # "/* Rysowanie ramki wokól znaku:\nDla znaku informacyjnego oraz nakazu i zakazu nalezy przeliczyc wspóBrzdne, wspóBrzdne ze skryptu Python mozna przekazac od razu do VI 'Overlay Rectangle'\nNIE JEST OBSLUGIWANE RYSOWANIE RAMKI WOKOL ZNAKU OSTRZEGAWCZEGO */"
        # "Template Separator\n(You can make a copy of, or modify, this frame)"
        n99 = Unbundle By Name(w307) -> ("Obraz"=w301:T1, "Rectangles"=w306:T6, "Circles"=w305:T7, "Znak"=w302:string, "Triangle"=w299:T4, "Python cords"=w303:T5)
        n100 = case shown="\"Znak informacyjny\"" w302 {
          tunnel: w306 -> [w314 _ _ _ _]
          tunnel: w305 -> [_ _ _ _ w320]
          tunnel: [w315 T5 {"Left"=0, "Top"=0, "Right"=0, "Bottom"=0} ("output cluster") w317 T5 {"Left"=0, "Top"=0, "Right"=0, "Bottom"=0} ("output cluster") w319] -> w304
          tunnel: w299 -> [_ _ _ _ _]
          tunnel: w303 -> [_ _ w317 _ _]
          frame "Znak informacyjny" {
            n101 = call "rectangleBox.vi"("Rectangles 2"=w314) -> ("output cluster"=w315:T5)
          }
          frame "Nie rozpoznano znaku !" {
          }
          frame "", Default {
          }
          frame "Znak ostrzegawczy" {
          }
          frame "Znak nakazu lub zakazu" {
            n102 = call "circleBox.vi"("Circles 3"=w320) -> ("output cluster"=w319:T5)
          }
        }
        n103 = call "IMAQ Overlay Rectangle"("Color"=u32 16711680, "error in (no error)"=w310, "Rectangle"=w304, "Image"=w301) -> ("error out"=w311:errorcluster, "Image Out"=w300:T1)  [unwired: 6 in]
        n104 = Bundle By Name(cluster=w307, "Obraz"=w300) -> (w308:T9)
        n105 = call <vilib>:"Add State(s) to Queue__JKI_lib_State_Machine.vi"("State(s) in (\"\")"=w313) -> ("States Out"=w312:string)  [unwired: 14 in]
      }
      frame "Action: Analyze Image" {
        w332 = 0 items=["Red", "Green", "Blue", "Hue", "Saturation", "Luminance", "Value", "Intensity"] ("Color Plane")
        w335 = T12 {"Rotation"=TRUE, "Scale"=TRUE, "Occlusion"=TRUE, "Range Settings"=[]} ("Match Options")
        # "/* Analiza poprzez funkcje LabView:\nDo analizy okregow i prostokatow wykorzystano\ngotowe VI Detect Shapes, do wykrywania trojkatow stworzono wlasny model wykrywania na podstawie templatu znajdujacego sie w folderze templates. Odczytany obraz przechodzi po kolei przez kazdy VI, a nastepnie w VI Detect Shapes odbywa sie porownanie informacji zwroconych przez kazde z VI oraz przekazanie nazwy znaku */"
        n106 = Unbundle By Name(w327) -> ("Obraz"=w339:T1)
        n107 = call "IMAQ Create"("Image Name"="analiza") -> ("New Image"=w338:T1)  [unwired: 4 in, 1 out]
        n108 = call "IMAQ Copy"("Image Dst"=w338, "Image Src"=w339) -> ("Image Dst Out"=w333:T1)  [unwired: 4 in, 1 out]
        n109 = call "IMAQ ExtractSingleColorPlane"("Color Plane"=w332, "Image Src"=w333) -> ("Image Dst Out"=w325:T1)  [unwired: 8 in, 1 out]
        n110 = call-poly "IMAQ Detect Shapes"("Match Options"=w335, "Rectangle Descriptor"=T8 {"Min Width"=40.0, "Max Width"=400.0, "Min Height"=40.0, "Max Height"=400.0}, "Image"=w325) -> ("Number of Matches Returned"=w331:i32, "Rectangles"=w329:T6)  [unwired: 6 in, 1 out]
        "Rectangles" <- w331
        n111 = call-poly "IMAQ Detect Shapes"("Minimum match score"=0.01, "error in (no error)"=w341, "Match Options"=w335, "Circle Descriptor"=cluster{"Min Radius":dbl, "Max Radius":dbl} {"Min Radius"=50.0, "Max Radius"=5000.0}, "Image"=w325) -> ("error out"=w342:errorcluster, "Number of Matches Returned"=w330:i32, "Circles"=w322:T7)  [unwired: 4 in]
        "Circles" <- w330
        n112 = call "traingleDet.vi"("Image"=w325) -> ("Number of Matches"=w324:i32, "Matches (pixel)"=w323:T4)  [unwired: 8 in, 1 out]
        "Triangles" <- w324
        n113 = call "detectShape.vi"("circle"=w330, "rectangle"=w331, "triangle"=w324) -> ("String"=w326:string)
        n114 = Bundle By Name(cluster=w327, "Rectangles"=w329, "Circles"=w322, "Znak"=w326, "Triangle"=w323, "L/p"="LabView") -> (w328:T9)
        n115 = call <vilib>:"Add State(s) to Queue__JKI_lib_State_Machine.vi"("State(s) in (\"\")"=w344) -> ("States Out"=w343:string)  [unwired: 14 in]
      }
      frame "Action: Load Image" {
        # "/* Zaladowanie zdjecia z danej sciazki z wykorzystaniem funkcji IMAQ */"
        # "Your code here.\n(You can make a copy of, or modify, this frame)"
        n116 = call "IMAQ GetFileInfo"("File Path"="Input Path") -> ("Image Type"=w351:T14)  [unwired: 4 in, 6 out]
        n117 = call "IMAQ Create"("Image Name"="image", "Image Type"=w351) -> ("New Image"=w350:T1)  [unwired: 3 in, 1 out]
        n118 = call "IMAQ ReadFile 2"("File Path"="Input Path", "Image"=w350) -> ("Image Out"=w348:T1)  [unwired: 5 in, 4 out]
        n119 = Bundle By Name(cluster=w346, "Obraz"=w348, "Input Path"="Input Path") -> (w347:T9)
        n120 = call <vilib>:"Add State(s) to Queue__JKI_lib_State_Machine.vi"("State(s) in (\"\")"=w354) -> ("States Out"=w353:string)  [unwired: 14 in]
      }
      frame "Action: Save Image" {
        # "/* Zapisywanie zdjecia w okrelsonej sciezka lokalizacji */"
        # "Your code here.\n(You can make a copy of, or modify, this frame)"
        n121 = Unbundle By Name(w356) -> ("Obraz"=w355:T1)
        n122 = call-poly "IMAQ Write File 2"("error in (no error)"=w358, "File Path"="Output Path", "Image"=w355) -> ("error out"=w359:errorcluster)  [unwired: 7 in, 1 out]
        n123 = call <vilib>:"Add State(s) to Queue__JKI_lib_State_Machine.vi"("State(s) in (\"\")"=w361) -> ("States Out"=w360:string)  [unwired: 14 in]
      }
      frame "Action: Clear Image" {
        # "/* Czyszczenie zdjecia oraz nazwy znaku na ekranie glownym */"
        # "Your code here.\n(You can make a copy of, or modify, this frame)"
        n124 = Bundle By Name(cluster=w364, "Obraz"=T1 refnum, "Znak"="") -> (w365:T9)
        n125 = call <vilib>:"Add State(s) to Queue__JKI_lib_State_Machine.vi"("State(s) in Front (\"\")"="UI: Update" ("State(s) in Front (\"\")"), "State(s) in (\"\")"=w369) -> ("States Out"=w368:string)  [unwired: 13 in]
      }
      frame "Action: SendToDataBase" {
        # "/* Przeslanie nazwy znaku wraz z rodzajem analizy do bazy danych */"
        n126 = call-poly <vilib>:"DB Tools Open Connection.vi"("error in (no error)"=w373, "connection information"="OSP") -> ("error out"=w387:errorcluster, "connection reference"=w388:T15)  [unwired: 6 in]
        n127 = Unbundle By Name(w381) -> ("Input Path"=w383:path)
        n128 = call <vilib>:"DB Tools Create Parameterized Query.vi"("error in (no error)"=w387, "SQL query"="insert into Recognized_images (Path,Category,Detection) values (?, ?, ?)", "connection reference"=w388) -> ("error out"=w391:errorcluster, "command reference"=w394:T16)  [unwired: 4 in, 1 out]
        n129 = Path To String(path=w383) -> (string=w382:string)
        n130 = call-poly <vilib>:"DB Tools Set Parameter Value.vi"("error in (no error)"=w391, "value"=w382, "parameter index"=0, "command reference"=w394) -> ("error out"=w393:errorcluster, "command reference out"=w392:T16)  [unwired: 4 in]
        n131 = Unbundle By Name(w381) -> ("Znak"=w384:string)
        n132 = call-poly <vilib>:"DB Tools Set Parameter Value.vi"("error in (no error)"=w393, "value"=w384, "parameter index"=1, "command reference"=w392) -> ("error out"=w378:errorcluster, "command reference out"=w379:T16)  [unwired: 4 in]
        n133 = Unbundle By Name(w381) -> ("L/p"=w380:string)
        n134 = call-poly <vilib>:"DB Tools Set Parameter Value.vi"("error in (no error)"=w378, "value"=w380, "parameter index"=2, "command reference"=w379) -> ("error out"=w376:errorcluster, "command reference out"=w377:T16)  [unwired: 4 in]
        n135 = call-poly <vilib>:"DB Tools Execute Query.vi"("error in (no error)"=w376, "command reference"=w377) -> ("error out"=w395:errorcluster, "command-recordset reference"=w396:T17)  [unwired: 6 in]
        n136 = call-poly <vilib>:"DB Tools Free Object.vi"("error in (no error)"=w395, "command-recordset reference"=w396) -> ("error out"=w390:errorcluster, "command reference"=w397:T16)  [unwired: 8 in]
        n137 = call-poly <vilib>:"DB Tools Free Object.vi"("error in (no error)"=w390, "command reference"=w397) -> ("error out"=w385:errorcluster, "connection reference"=w386:T15)  [unwired: 8 in]
        n138 = call <vilib>:"DB Tools Close Connection.vi"("error in (no error)"=w385, "connection reference"=w386) -> ("error out"=w398:errorcluster)  [unwired: 5 in]
        n139 = call <vilib>:"Simple Error Handler.vi"("error in (no error)"=w398) -> ("error out"=w374:errorcluster)  [unwired: 4 in, 4 out]
        n140 = call <vilib>:"Add State(s) to Queue__JKI_lib_State_Machine.vi"("State(s) in (\"\")"=w400) -> ("States Out"=w399:string)  [unwired: 14 in]
      }
    }
  }
